vi "Simpson Test.vi"() -> ()   [LabVIEW 2017]
panel:
  out "Value of Integral":dbl
  in  "Digitizing Parameters":T1={"Number of Samples"=100, "Lower Limit"=0.0, "Upper Limit"=1.0}
  in  "Function Parameters":cluster{"Prefactor":dbl, "Power":dbl}={"Prefactor"=5.0, "Power"=4.0}
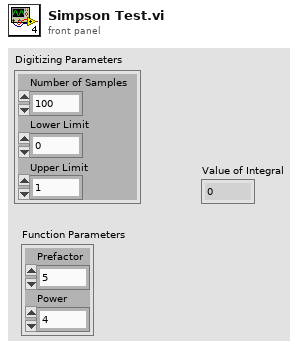
[diagram p1: front panel]
types:
  T1 = cluster{"Number of Samples":i32, "Lower Limit":dbl, "Upper Limit":dbl}
  T2 = cluster{"X Array":dbl[], "Y Array":dbl[], "delta_x":dbl}
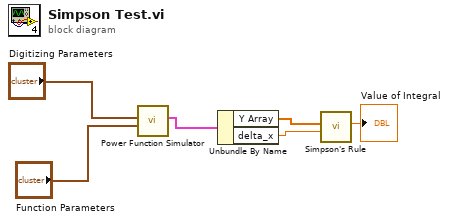
[diagram p0: block diagram]
diagram:
  n1 = call "Power Function Simulator.vi"("Function Parameters"="Function Parameters", "Digitizing Parameters"="Digitizing Parameters") -> ("Output Cluster"=w4:T2)  [unwired: 9 in]
  n2 = Unbundle By Name(w4) -> ("Y Array"=w3:dbl[], "delta_x"=w2:dbl)
  n3 = call "Simpson's Rule.vi"("delta_x"=w2, "Array"=w3) -> ("Value of Integral"=→"Value of Integral":dbl)  [unwired: 9 in]
